vi "Array to Offset and Multiplier.vi"(1 "Array":dbl[](array[numeric])) -> (0 "Offset and Multiplier":T1)   [LabVIEW 2016, in "Tranconductance SM.lvclass"]
doc: "Given an array, calculate an Offset and Multiplier"
uses:
  Tranconductance SM.lvclass
  <vilib>/Utility/miscctls.llb/LVOffsetAndMultiplierTypeDef.ctl
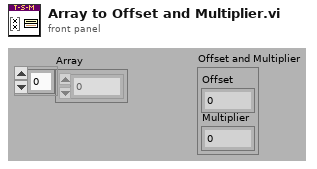
[diagram p1: front panel]
types:
  T1 = typedef "LVOffsetAndMultiplierTypeDef.ctl" = cluster{"Offset":dbl, "Multiplier":dbl}
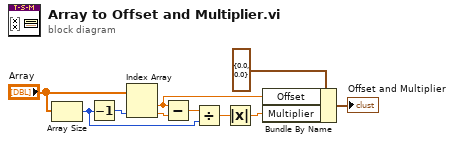
[diagram p0: block diagram]
diagram:
  n1 = Array Size(array="Array") -> (size(s)=w3:i32)
  n2 = Decrement(x=w3) -> (x-1=w5:i32)
  n3 = Index Array(array="Array", index #2=w5) -> (element #1=w10:dbl, element #2=w9:dbl)  [unwired: 1 in]
  n4 = Subtract(x=w10, y=w9) -> (x-y=w4:dbl)
  n5 = Divide(x=w4, y=w3) -> (x/y=w2:dbl)
  n6 = Absolute Value(x=w2) -> (abs(x)=w1:dbl)
  n7 = Bundle By Name(cluster=T1 {"Offset"=0.0, "Multiplier"=0.0} ("X Scale.Offset and Multiplier"), "Offset"=w10, "Multiplier"=w1) -> (→"Offset and Multiplier":T1)
